vi "fun_ParametersToPaths&Values.vi"(10 "Parameters":T1[](array[typedef]) {"Value" format="%#_6p"}) -> (1 "Values":dbl[](array[numeric]), 2 "Paths":string[](array[string]))   [LabVIEW 2016, in "General.lvlib"]
uses:
  General.lvlib
  Ctl_SetParameter(Value).ctl
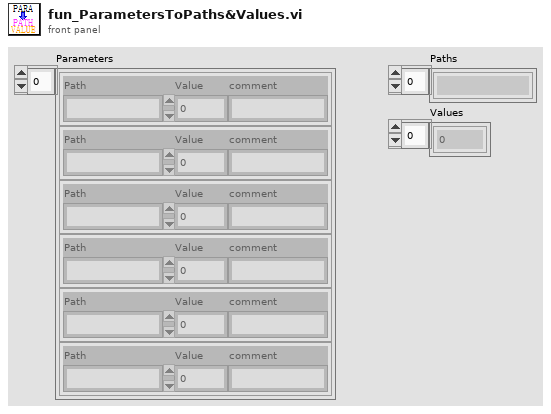
[diagram p1: front panel]
types:
  T1 = typedef "General.lvlib/Ctl_SetParameter(Value).ctl" = cluster{"Path":string, "Value":dbl, "comment":string}
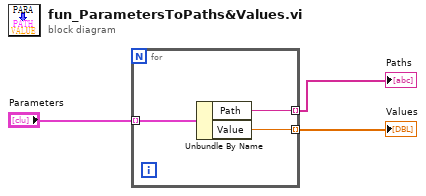
[diagram p0: block diagram]
diagram:
  n1 = for {
    tunnel: "Parameters" -> [w6] mode=indexing
    tunnel: [w5] -> w2 mode=indexing
    tunnel: [w4] -> w1 mode=indexing
    n2 = Unbundle By Name(w6) -> ("Path"=w5:string, "Value"=w4:dbl)
  }
  "Paths" <- w2
  "Values" <- w1
